vi "Off.vi"(8 "error in (no error)":errorcluster, 11 "reference in":refnum<class "CeilingFan.lvclass">) -> (0 "error out":errorcluster, 3 "reference out":refnum<class "CeilingFan.lvclass">)   [LabVIEW 2020, in "CeilingFan.lvclass"]
uses:
  CeilingFan.lvclass
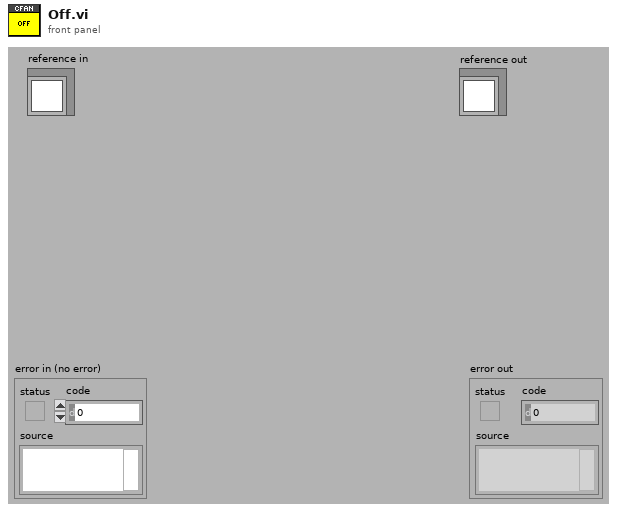
[diagram p1: front panel]
types:
  T1 = typedef "CeilingFan.lvclass/ObjectAttributes.ctl" = cluster{"Speed":i32}
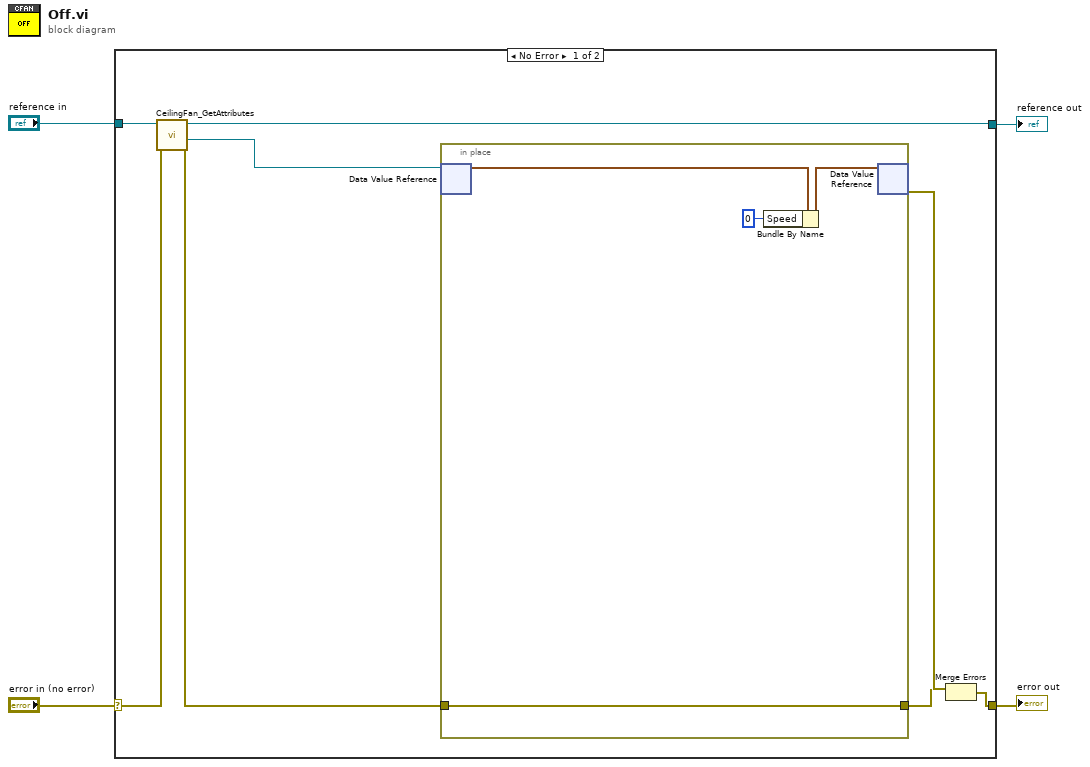
[diagram p0: block diagram]
diagram:
  n1 = case shown="No Error" "error in (no error)" {
    selector: "error in (no error)" -> [w11 w18]
    tunnel: [w8 w18] -> w3
    tunnel: [w9 w17] -> w1
    tunnel: "reference in" -> [w12 w17]
    frame No Error {
      n2 = call "CeilingFan_GetAttributes.vi"("error in (no error)"=w11, "reference in"=w12) -> ("error out"=w6:errorcluster, "DataRef"=w7:refnum<data-value>, "reference out"=w9:refnum<class "CeilingFan.lvclass">)  [unwired: 6 in, 1 out]
      n3 = in-place {
        in-place-border: w6 -> [w15]
        in-place-border: [w15] -> w5
        n4 = in-place-dvr #1(w7) -> (w14:T1)  [unwired: 1 out]
        n5 = Bundle By Name(cluster=w14, "Speed"=0) -> (w16:T1)
        n6 = in-place-dvr #1(w16) -> (w10:errorcluster)  [unwired: 1 out]
      }
      n7 = Merge Errors(w10, w5) -> (w8:errorcluster)
    }
    frame Error {
    }
  }
  "error out" <- w3
  "reference out" <- w1
